vi "Read TDMS XYN.vi"(8 "error in (no error)":errorcluster, 9 "Channels":cluster{"X":string, "Y":string, "N":string}, 10 "File or Folder Path":path=path "C:/", 11 "LVtoITX.lvclass":refnum<class "LV to ITX.lvclass">) -> (0 "error out":errorcluster, 1 "N []":dbl[](array[numeric]), 2 "Y vs X []":cluster{dbl[], dbl[]}[](graph), 3 "LVtoITX.lvclass out":refnum<class "LV to ITX.lvclass">)   [LabVIEW 2016, in "LV to ITX.lvclass"]
uses:
  LV to ITX.lvclass
panel:
  out "Path":path
  in  "length":i32=1
  out "counter":i32
  in  "offset":i32
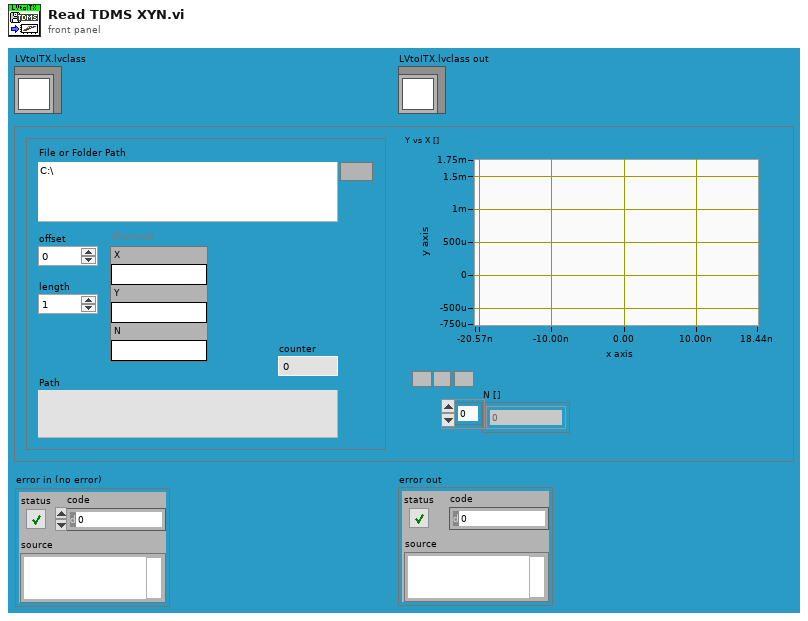
[diagram p1: front panel]
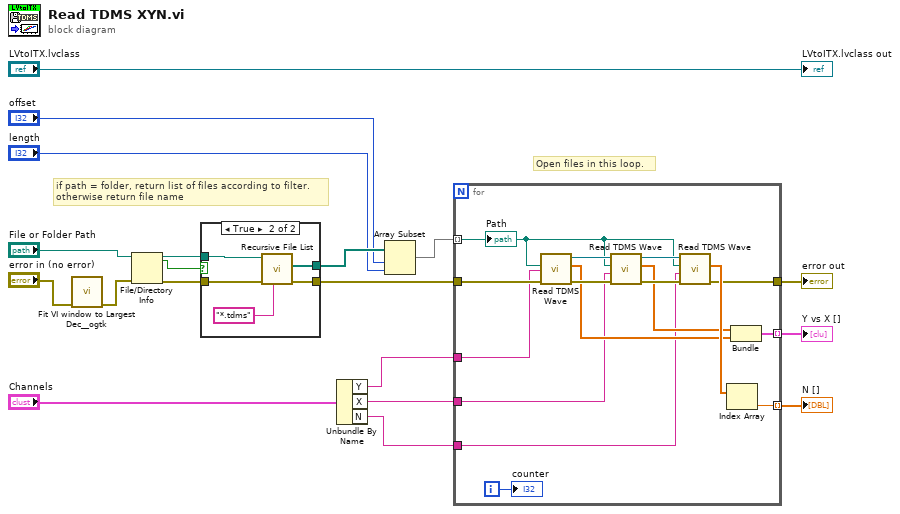
[diagram p0: block diagram]
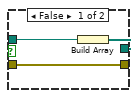
[diagram p2: hidden frame]
diagram:
  # "Open files in this loop."
  # "if path = folder, return list of files according to filter.\notherwise return file name"
  n1 = call <userlib>:"Fit VI window to Largest Dec__ogtk.vi"("error in (no error)"="error in (no error)") -> ("error out"=w9:errorcluster)  [unwired: 5 in, 1 out]
  n2 = File/Directory Info(path="File or Folder Path", error in=w9) -> (path out=w12:path, directory=w14:bool, error out=w13:errorcluster)  [unwired: 4 out]
  n3 = case shown="True" w14 {
    tunnel: [w22 w26] -> w19
    tunnel: w12 -> [w21 w27]
    tunnel: w13 -> [w20 w25]
    tunnel: [w20 w24] -> w15
    frame False {
      n4 = Build Array(w21) -> (w22:path[])
    }
    frame True {
      n5 = call <vilib>:"Recursive File List.vi"("pattern"="*.tdms", "error in (no error)"=w25, "Folder Path"=w27) -> ("error out"=w24:errorcluster, "All Files in Dir"=w26:path[])  [unwired: 4 in, 3 out]
    }
  }
  n6 = Unbundle By Name("Channels") -> ("Y"=w8:string, "X"=w7:string, "N"=w6:string)
  n7 = Array Subset(array=w19, index="offset", length="length") -> (w2:path[])
  n8 = for {
    tunnel: w2 -> [w34] mode=indexing
    tunnel: [w42] -> w1 mode=indexing
    tunnel: w15 -> [w41]
    tunnel: [w35] -> w4 mode=indexing
    tunnel: [w33] -> w5
    tunnel: w8 -> [w30]
    tunnel: w7 -> [w29]
    tunnel: w6 -> [w28]
    i -> [w43]
    n9 = call "Read TDMS Wave.vi"("error in (no error)"=w41, "channel name(s) in"=w30, "path"=w34) -> ("error out"=w40:errorcluster, "data"=w31:dbl[], "LVtoITX out"=w39:refnum<class "LV to ITX.lvclass">)  [unwired: 6 in]
    n10 = call "Read TDMS Wave.vi"("error in (no error)"=w40, "channel name(s) in"=w29, "path"=w34, "LVtoITX in"=w39) -> ("error out"=w38:errorcluster, "data"=w32:dbl[], "LVtoITX out"=w37:refnum<class "LV to ITX.lvclass">)  [unwired: 5 in]
    n11 = call "Read TDMS Wave.vi"("error in (no error)"=w38, "channel name(s) in"=w28, "path"=w34, "LVtoITX in"=w37) -> ("error out"=w33:errorcluster, "data"=w36:dbl[])  [unwired: 5 in, 1 out]
    n12 = Index Array(array=w36) -> (element=w35:dbl)  [unwired: 1 in]
    n13 = Bundle("data"=w32, "data"=w31) -> (w42:cluster{"data":dbl[], "data":dbl[]})  [unwired: 1 in]
    "counter" <- w43
    "Path" <- w34
  }
  "error out" <- w5
  "Y vs X []" <- w1
  "N []" <- w4
  "LVtoITX.lvclass out" <- "LVtoITX.lvclass"
